vi "FGV_NewTable.vi"(7 "GET_SET":T1, 11 "Prop in":T2={"Table_Name"="", "Column Info"=[{"column name"="Signal_x", "data type"=enum."Double (DBL)", "size"=0, "allow null?"=TRUE}, {"column name"="Signal_y", "data type"=enum."Double (DBL)", "size"=0, "allow null?"=TRUE}, {"column name"="Signal_z", "data type"=enum."Double (DBL)", "size"=0, "allow null?"=TRUE}], "ColumnNames"=[]}) -> (3 "Prop out":T2={"Table_Name"="", "Column Info"=[{"column name"="Signal_x", "data type"=enum."Double (DBL)", "size"=0, "allow null?"=TRUE}, {"column name"="Signal_y", "data type"=enum."Double (DBL)", "size"=0, "allow null?"=TRUE}, {"column name"="Signal_z", "data type"=enum."Double (DBL)", "size"=0, "allow null?"=TRUE}], "ColumnNames"=[]})   [LabVIEW 2019]
uses:
  TypeDef/#TypeDef_NewTable.ctl
  <vilib>/addons/database/Auxilliary.llb/DB Tools Column Info.ctl
  <vilib>/addons/database/Auxilliary.llb/DB Tools DataTypes.ctl
  TypeDef/#TypeDef_GET_SET.ctl
  <vilib>/addons/database/NI_Database_API.lvlib
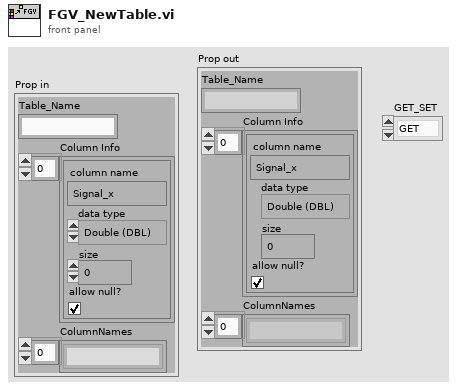
[diagram p1: front panel]
types:
  T1 = typedef "#TypeDef_GET_SET.ctl" = enum16{"GET", "SET"}
  T2 = typedef "#TypeDef_NewTable.ctl" = cluster{"Table_Name":string, "Column Info":T3[], "ColumnNames":string[]}
  T3 = typedef "NI_Database_API.lvlib/DB Tools Column Info.ctl" = cluster{"column name":string, "data type":T4, "size":i32, "allow null?":bool}
  T4 = typedef "NI_Database_API.lvlib/DB Tools DataTypes.ctl" = enum16{"String", "Long (I32)", "Single (SGL)", "Double (DBL)", "Date/Time", "Binary"}
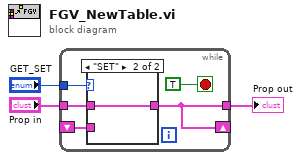
[diagram p0: block diagram]
diagram:
  n1 = while {
    tunnel: "GET_SET" -> [w8]
    tunnel: "Prop in" -> [w7]
    tunnel: [w6] -> w3
    shift-right: [w6] -> _
    shift-left: _ -> [w5]
    stop <- TRUE stop-if-true
    n2 = case shown="\"SET\"" w8 {
      tunnel: w7 -> [_ w10]
      tunnel: [w9 w10] -> w6
      tunnel: w5 -> [w9 _]
      frame "GET", Default {
      }
      frame "SET" {
      }
    }
  }
  "Prop out" <- w3
